vi "Set Theme.vi"(10 "Dark?":bool, 11 "VI in":refnum<vi>) -> ()   [LabVIEW 2019, in "Panther Dashboard.lvlib"]
uses:
  Panther Dashboard.lvlib
  <vilib>/Utility/miscctls.llb/LVTextColorsTypeDef.ctl
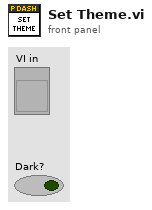
[diagram p1: front panel]
types:
  T1 = typedef "LVTextColorsTypeDef.ctl" = cluster{"Text Color":u32, "Background Color":u32}
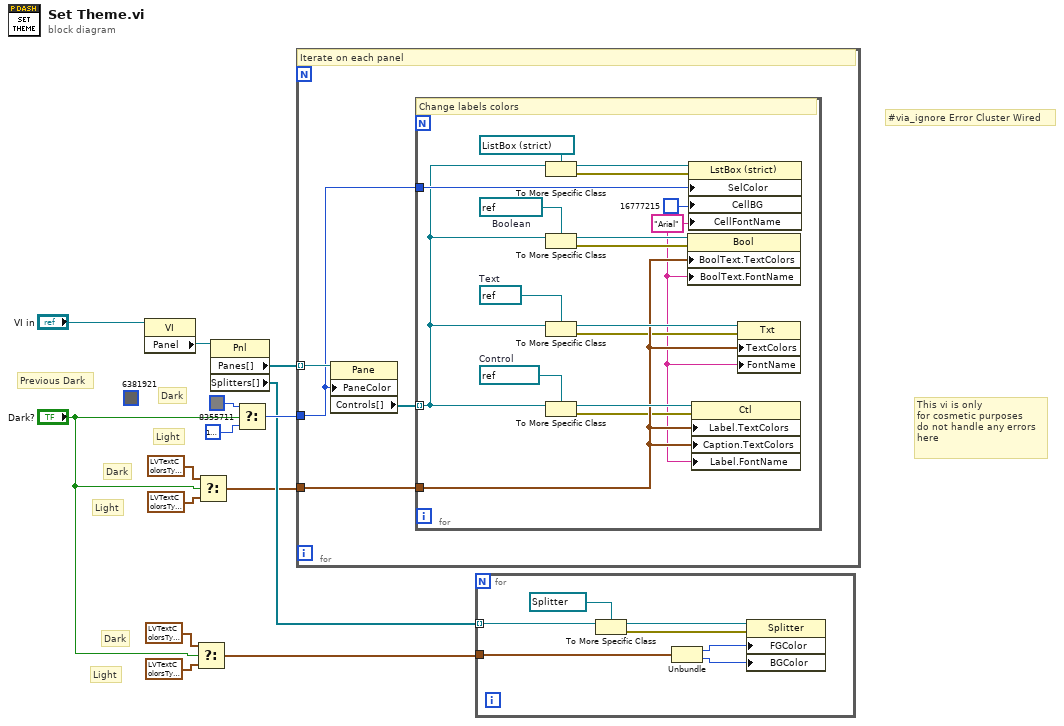
[diagram p0: block diagram]
diagram:
  (unwired) u32 6381921
  # "Previous Dark"
  # "Light"
  # "Dark"
  # "Light"
  # "Dark"
  # "#via_ignore Error Cluster Wired"
  # "This vi is only \nfor cosmetic purposes\ndo not handle any errors\nhere"
  # "Light"
  # "Dark"
  n1 = property class="VI"(reference="VI in") -> ("Panel"=w10:refnum<vi>)  [unwired: 1 in, 2 out]
  n2 = Select(t=T1 {"Text Color"=9145227, "Background Color"=16448250} ("Label.Text Colors"), s="Dark?", f=T1 {"Text Color"=14540253, "Background Color"=13816530} ("Label.Text Colors")) -> (s? t:f=w3:T1)
  n3 = Select(t=T1 {"Text Color"=16448250, "Background Color"=16777216} ("Label.Text Colors"), s="Dark?", f=T1 {"Text Color"=0, "Background Color"=16777216} ("Label.Text Colors")) -> (s? t:f=w6:T1)
  n4 = property class="Pnl"(reference=w10) -> ("Panes[]"=w9:refnum<vi>[], "Splitters[]"=w7:refnum<vi>[])  [unwired: 1 in, 2 out]
  n5 = Select(t=u32 8355711, s="Dark?", f=u32 16777238) -> (s? t:f=w8:u32)
  n6 = for {
    tunnel: w9 -> [w17] mode=indexing
    tunnel: w8 -> [w15]
    tunnel: w6 -> [w18]
    # "Iterate on each panel"
    n7 = property class="Pane"(reference=w17, "PaneColor"=w15) -> ("Controls[]"=w16:refnum<vi>[])  [unwired: 1 in, 2 out]
    n8 = for {
      tunnel: w16 -> [w26] mode=indexing
      tunnel: w18 -> [w25]
      tunnel: w15 -> [w27]
      w19 = "Arial" ("Active Row:Cell Font:Name")
      w31 = refnum<vi> refnum  # Boolean
      w32 = refnum<vi> refnum  # Text
      w34 = refnum<vi> refnum  # Control
      # "Change labels colors"
      n9 = To More Specific Class(target class=refnum<vi> refnum ("Projects 2"), reference=w26) -> (specific class reference=w28:refnum<vi>, error out=w24:errorcluster)  [unwired: 1 in]
      n10 = To More Specific Class(target class=w31, reference=w26) -> (specific class reference=w30:refnum<vi>, error out=w23:errorcluster)  [unwired: 1 in]
      n11 = To More Specific Class(target class=w32, reference=w26) -> (specific class reference=w33:refnum<vi>, error out=w22:errorcluster)  [unwired: 1 in]
      n12 = To More Specific Class(target class=w34, reference=w26) -> (specific class reference=w35:refnum<vi>, error out=w21:errorcluster)  [unwired: 1 in]
      n13 = property class="Bool"(reference=w30, error in=w23, "BoolText.TextColors"=w25, "BoolText.FontName"=w19) -> ()  [unwired: 2 out]
      n14 = property class="LstBox (strict)"(reference=w28, error in=w24, "SelColor"=w27, "CellBG"=u32 16777215, "CellFontName"=w19) -> ()  [unwired: 2 out]
      n15 = property class="Ctl"(reference=w35, error in=w21, "Label.TextColors"=w25, "Caption.TextColors"=w25, "Label.FontName"=w19) -> ()  [unwired: 2 out]
      n16 = property class="Txt"(reference=w33, error in=w22, "TextColors"=w25, "FontName"=w19) -> ()  [unwired: 2 out]
    }
  }
  n17 = for {
    tunnel: w7 -> [w39] mode=indexing
    tunnel: w3 -> [w38]
    n18 = To More Specific Class(target class=refnum<vi> refnum ("Projects 2"), reference=w39) -> (specific class reference=w41:refnum<vi>, error out=w40:errorcluster)  [unwired: 1 in]
    n19 = Unbundle(w38) -> ("Text Color"=w37:u32, "Background Color"=w36:u32)
    n20 = property class="Splitter"(reference=w41, error in=w40, "FGColor"=w37, "BGColor"=w36) -> ()  [unwired: 2 out]
  }
